vi "Async Forwarding VI I32.vi"(9 "subchannel another channel (0)":i32, 10 "subchannel (0)":i32, 11 "channel":T1) -> (3 "another channel":T1)   [LabVIEW 2020, in "Tests Event MessengerM.lvclass"]
uses:
  Tests Event MessengerM.lvclass
  Tests Event MessengerM.lvclass/Tests Event MessengerM.ctl
  25f11a8f-d5bb-42c9-8e5c-05bf9bae4858.vi
  ba5f48a0-187d-4afe-82e9-726c0ace0d13.vi
  <extravilib>/ChannelInstances/Event MessengerM-i32/))Channel.ctl
  <extravilib>/ChannelInstances/Event MessengerM-i32.lvlib
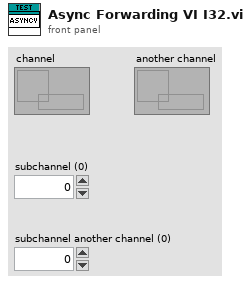
[diagram p1: front panel]
types:
  T1 = typedef "Event MessengerM-i32.lvlib/))Channel.ctl" = refnum<queue>
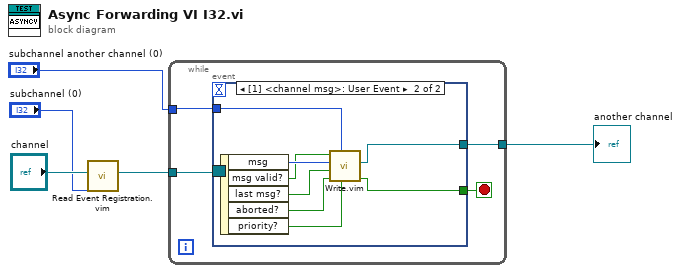
[diagram p0: block diagram]
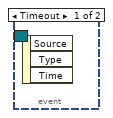
[diagram p2: hidden frame]
diagram:
  n1 = call "Read Event Registration.vim"("subchannel"="subchannel (0)", "channel"="channel") -> ("event registration refnum"=w4:refnum<event-registration>)  [unwired: 9 in]
  n2 = while {
    tunnel: w4 -> [w9]
    tunnel: "subchannel another channel (0)" -> [w7]
    tunnel: [w6] -> w3
    stop <- w8 stop-if-true
    n3 = event shown="[1] <channel msg>: User Event" {
      selector: w9 -> [_ _]
      dyn-events: _ -> [_ _]
      timeout: _ -> [_ _]
      tunnel: [_ w11] -> w8
      tunnel: w7 -> [_ w16]
      tunnel: [_ w10] -> w6
      event Timeout {
        n4 = event-data() -> ()  [unwired: 1 in, 3 out]
      }
      event User Event {
        n5 = event-data() -> ("msg"=w17:i32, "msg valid?"=w15:bool, "last msg?"=w14:bool, "aborted?"=w13:bool, "priority?"=w12:bool)  [unwired: 1 in]
        n6 = call "Write.vim"("high priority? (F)"=w12, "subchannel"=w16, "abort sub (F)"=w13, "last message? (F)"=w14, "element"=w17, "message valid? (T)"=w15) -> ("done?"=w11:bool, "channel"=w10:T1)  [unwired: 4 in]
      }
    }
  }
  "another channel" <- w3
